vi "configure_channel_ASIC.vi"() -> ()   [LabVIEW 2009]
panel:
  in  "Clip_sel_b":u32=2
  in  "Att_en_b":bool
  in  "Clip_en_b":bool
  in  "CompBuf_en_b":bool
  in  "Ib_ClipVb":u32=20
  in  "Att gain":u32=7
  out "written data":u32=72
  in  "Channel":u16(ring)=4 items=["Channel 0", "Channel 1", "Channel 2", "Channel 3", "Channel 4", "Channel 5", "Channel 6"]
  in  "Id in":u32
  out "total cycles":i32
  out "data read value":u32=72
  out "error out 2":errorcluster
  in  "error in (no error)":errorcluster
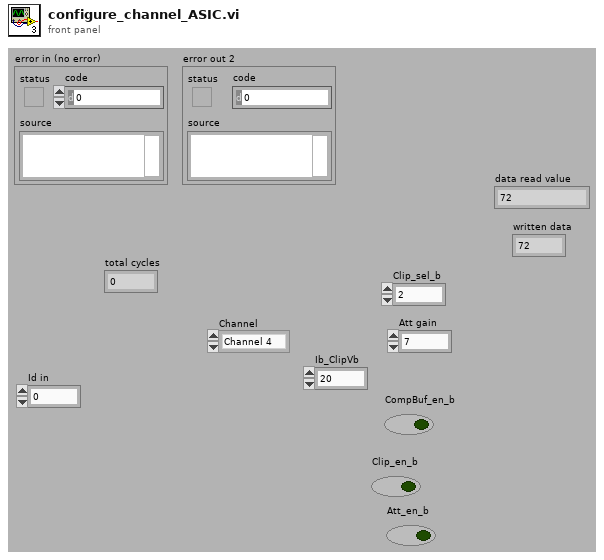
[diagram p1: front panel]
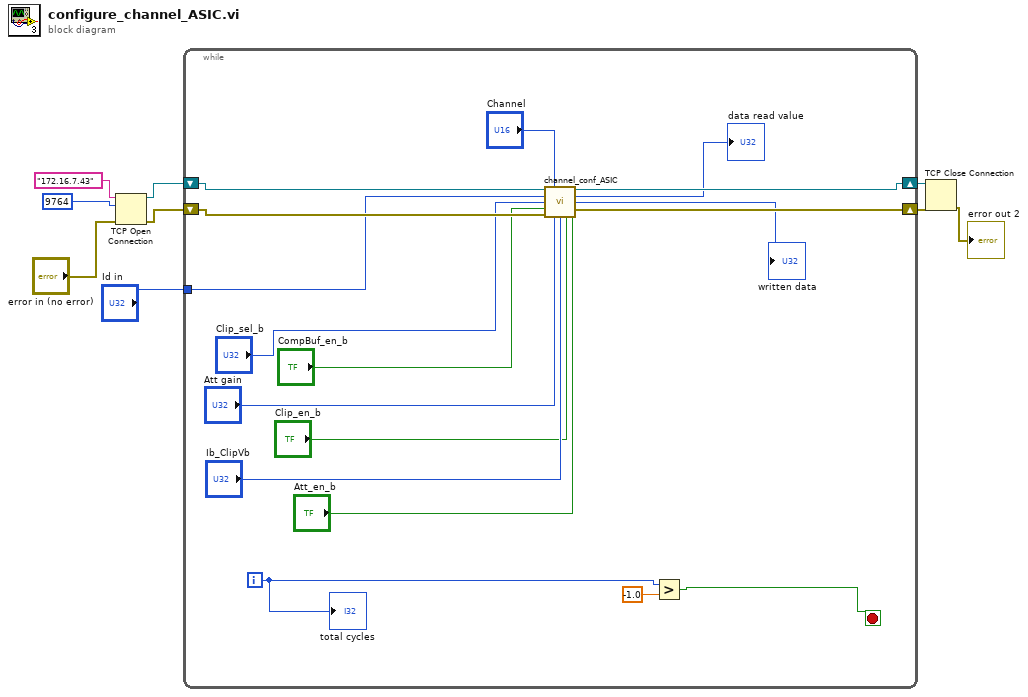
[diagram p0: block diagram]
diagram:
  n1 = TCP Open Connection(address="172.16.7.43", remote port or service name=u16 9764, error in (no error)="error in (no error)") -> (connection ID=w5:refnum<k5>, error out=w4:errorcluster)  [unwired: 2 in]
  n2 = while {
    shift-right: [w24] -> w7
    shift-left: w4 -> [w26]
    shift-right: [w23] -> w6
    shift-left: w5 -> [w25]
    tunnel: "Id in" -> [w12]
    i -> [w19]
    stop <- w21 stop-if-true
    n3 = call "channel_conf_ASIC.vi"("connection ID"=w25, "Ring"="Channel", "Id in"=w12, "Clip_sel_b"="Clip_sel_b", "CompBuf_en_b"="CompBuf_en_b", "error out"=w26, "Att gain"="Att gain", "Ib_ClipVb"="Ib_ClipVb", "Clip_en_b"="Clip_en_b", "Att_en_b"="Att_en_b") -> ("connection ID out"=w23:refnum<k5>, "data read value"=→"data read value":u32, "written data"=→"written data":u32, "error out 2"=w24:errorcluster)  [unwired: 1 in, 1 out]
    n4 = Greater?(x=w19, y=-1.0) -> (0:w21:bool)
    "total cycles" <- w19
  }
  n5 = TCP Close Connection(connection ID=w6, error in (no error)=w7) -> (error out=→"error out 2":errorcluster)  [unwired: 1 in, 1 out]
